vi "test_scd_GetLastError.vi"(8 "error in":errorcluster, 11 "SCD in":refnum<class "SCD.lvclass">) -> (0 "error out":errorcluster, 3 "SCD out":refnum<class "SCD.lvclass">)   [LabVIEW 2023, in "horiba.test.lvlib"]
uses:
  horiba.test.lvlib
  Classes/SCD/SCD.lvclass
  C:/Projects/Horiba/horiba-labview-sdk/Source/Classes/GenericDevice/GenericDevice.lvclass
  <vilib>/addons/_JKI Toolkits/Caraya/classes/Test/Test.lvclass
  <vilib>/addons/_JKI Toolkits/Caraya/classes/Assert/Assert.lvclass
  <userlib>/_OpenG.lib/lvdata/lvdata.llb/openg_variant.lvlib
  <vilib>/addons/_JKI Toolkits/Caraya/classes/Assert/Assert Not Equal Value_Variant.vi
panel:
  # "Connector Pane"
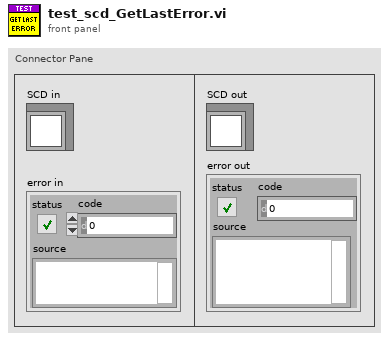
[diagram p1: front panel]
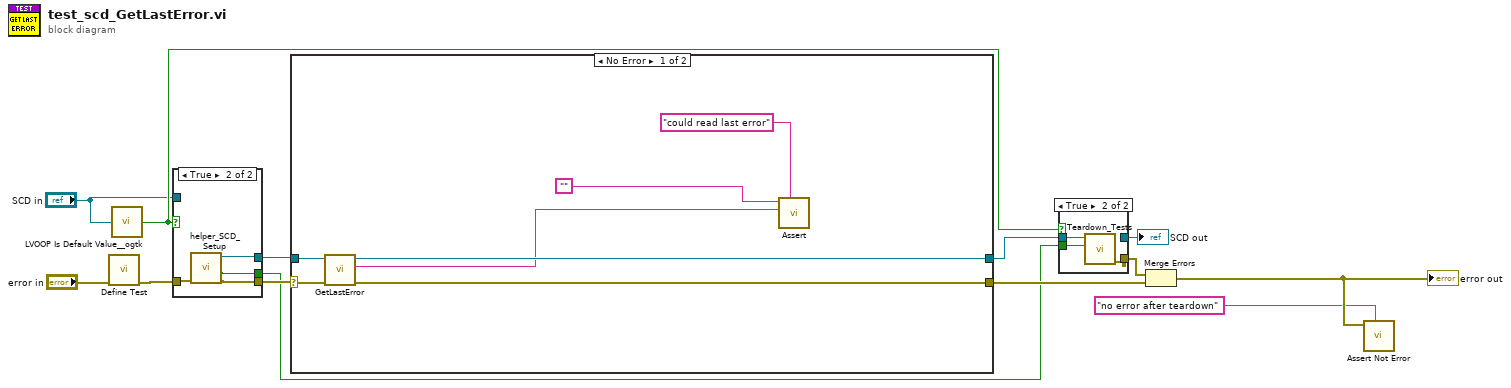
[diagram p0: block diagram]
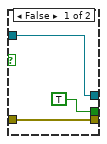
[diagram p3: hidden frame]
diagram:
  n1 = call <vilib>:"Define Test.vi"("error in (no error)"="error in") -> ("error out"=w9:errorcluster)  [unwired: 9 in, 1 out]
  n2 = call <userlib>:"LVOOP Is Default Value__ogtk.vi"("Object"="SCD in") -> ("Is Default Value?"=w3:bool)
  n3 = case shown="True" w3 {
    tunnel: w9 -> [w16 w18]
    tunnel: [w16 w20] -> w8
    tunnel: [w14 w17] -> w7
    tunnel: [TRUE ("Module Was Already Running?") w19] -> w4
    tunnel: "SCD in" -> [w14 _]
    frame False {
    }
    frame True {
      n4 = call "helper_SCD_Setup.vi"("error in"=w18) -> ("error out"=w20:errorcluster, "Module Was Already Running?"=w19:bool, "SCD out"=w17:refnum<class "SCD.lvclass">)  [unwired: 7 in, 1 out]
    }
  }
  n5 = case shown="No Error" w8 {
    selector: w8 -> [w26 w29]
    tunnel: [w24 w28] -> w12
    tunnel: w7 -> [w27 w28]
    tunnel: [w23 w29] -> w11
    frame No Error {
      n6 = call "GetLastError.vi"("error in (no error)"=w26, "SCD in"=w27) -> ("error out"=w23:errorcluster, "last_error"=w22:string, "SCD out"=w24:refnum<class "SCD.lvclass">)  [unwired: 7 in]
      n7 = call-poly <vilib>:"Assert.vi"("Label"="could read last error", "Y"=w22, "X"="") -> ()  [unwired: 7 in, 2 out]
    }
    frame Error {
    }
  }
  n8 = case shown="True" w3 {
    tunnel: w12 -> [w30 w33]
    tunnel: [_ w32] -> w6
    tunnel: w4 -> [_ w31]
    tunnel: [w30 _] -> w1
    frame False {
    }
    frame True {
      n9 = call "Teardown_Tests.vi"("Module Was Already Running?"=w31, "horiba.lvlib:GenericDevice"=w33) -> ("error out"=w32:errorcluster)  [unwired: 8 in, 1 out]
    }
  }
  "SCD out" <- w1
  n10 = Merge Errors(w6, w11) -> (w10:errorcluster)
  "error out" <- w10
  n11 = call <vilib>:"Assert Not Error.vi"("Label"="no error after teardown", "Not Error?"=w10) -> ()  [unwired: 8 in, 2 out]
